vi "main_array.vi"() -> ()   [LabVIEW 2017]
panel:
  out "Numeric":i32
  out "error out":errorcluster
  in  "stop":bool
  in  "Mode":T1(tab)
  out "Polar Plot":picture
  in  "Plot Color":u32(colorbox)=16715776
  in  "Grid Color":u32(colorbox)
  in  "Visible Section":u16(ring)=8
  out "Range":dbl(slide) scale=0.0..600.0
  out "Histogram":picture
  in  "Clear":bool
  out "Array":i32[](array[numeric])
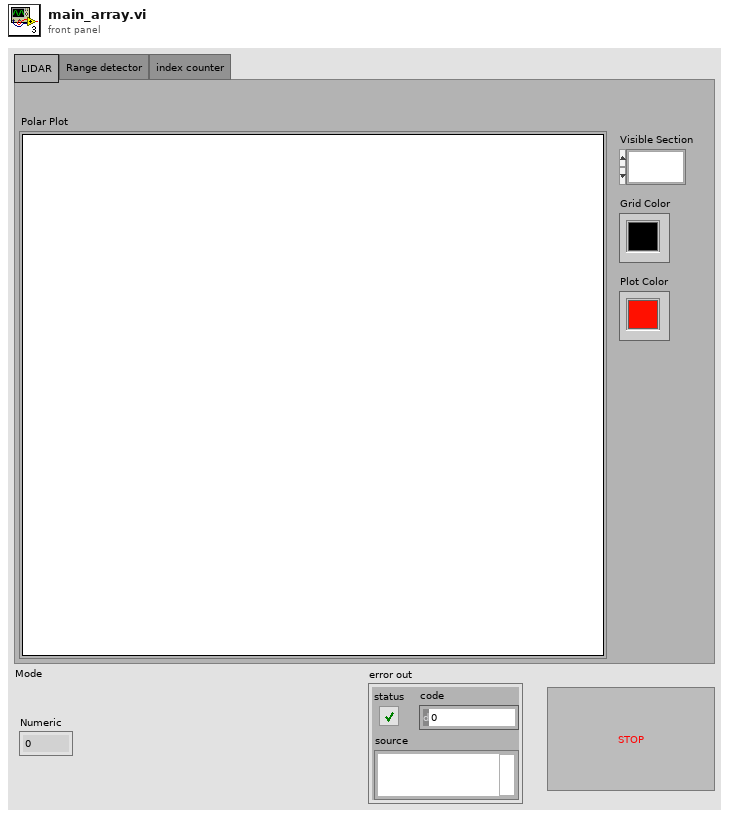
[diagram p1: front panel]
types:
  T1 = enum32{"LIDAR", "Range detector", "index counter"}
  T2 = cluster{"maximum":dbl, "minimum":dbl, "clip to min":bool, "log?(F)":bool, "grid color":u32, "plot color":u32, "format and precision":cluster{"format":enum8{"Decimal", "Scientific", "Engineering", "Binary", "Octal", "Hex"}, "precision":u8}, "visible section":u16}
  T3 = typedef "LVBoundsTypeDef.ctl" = cluster{"Width":u32, "Height":u32}
  T4 = cluster{"distance (C/AI0 (AI0))":dbl, "Numeric":dbl}
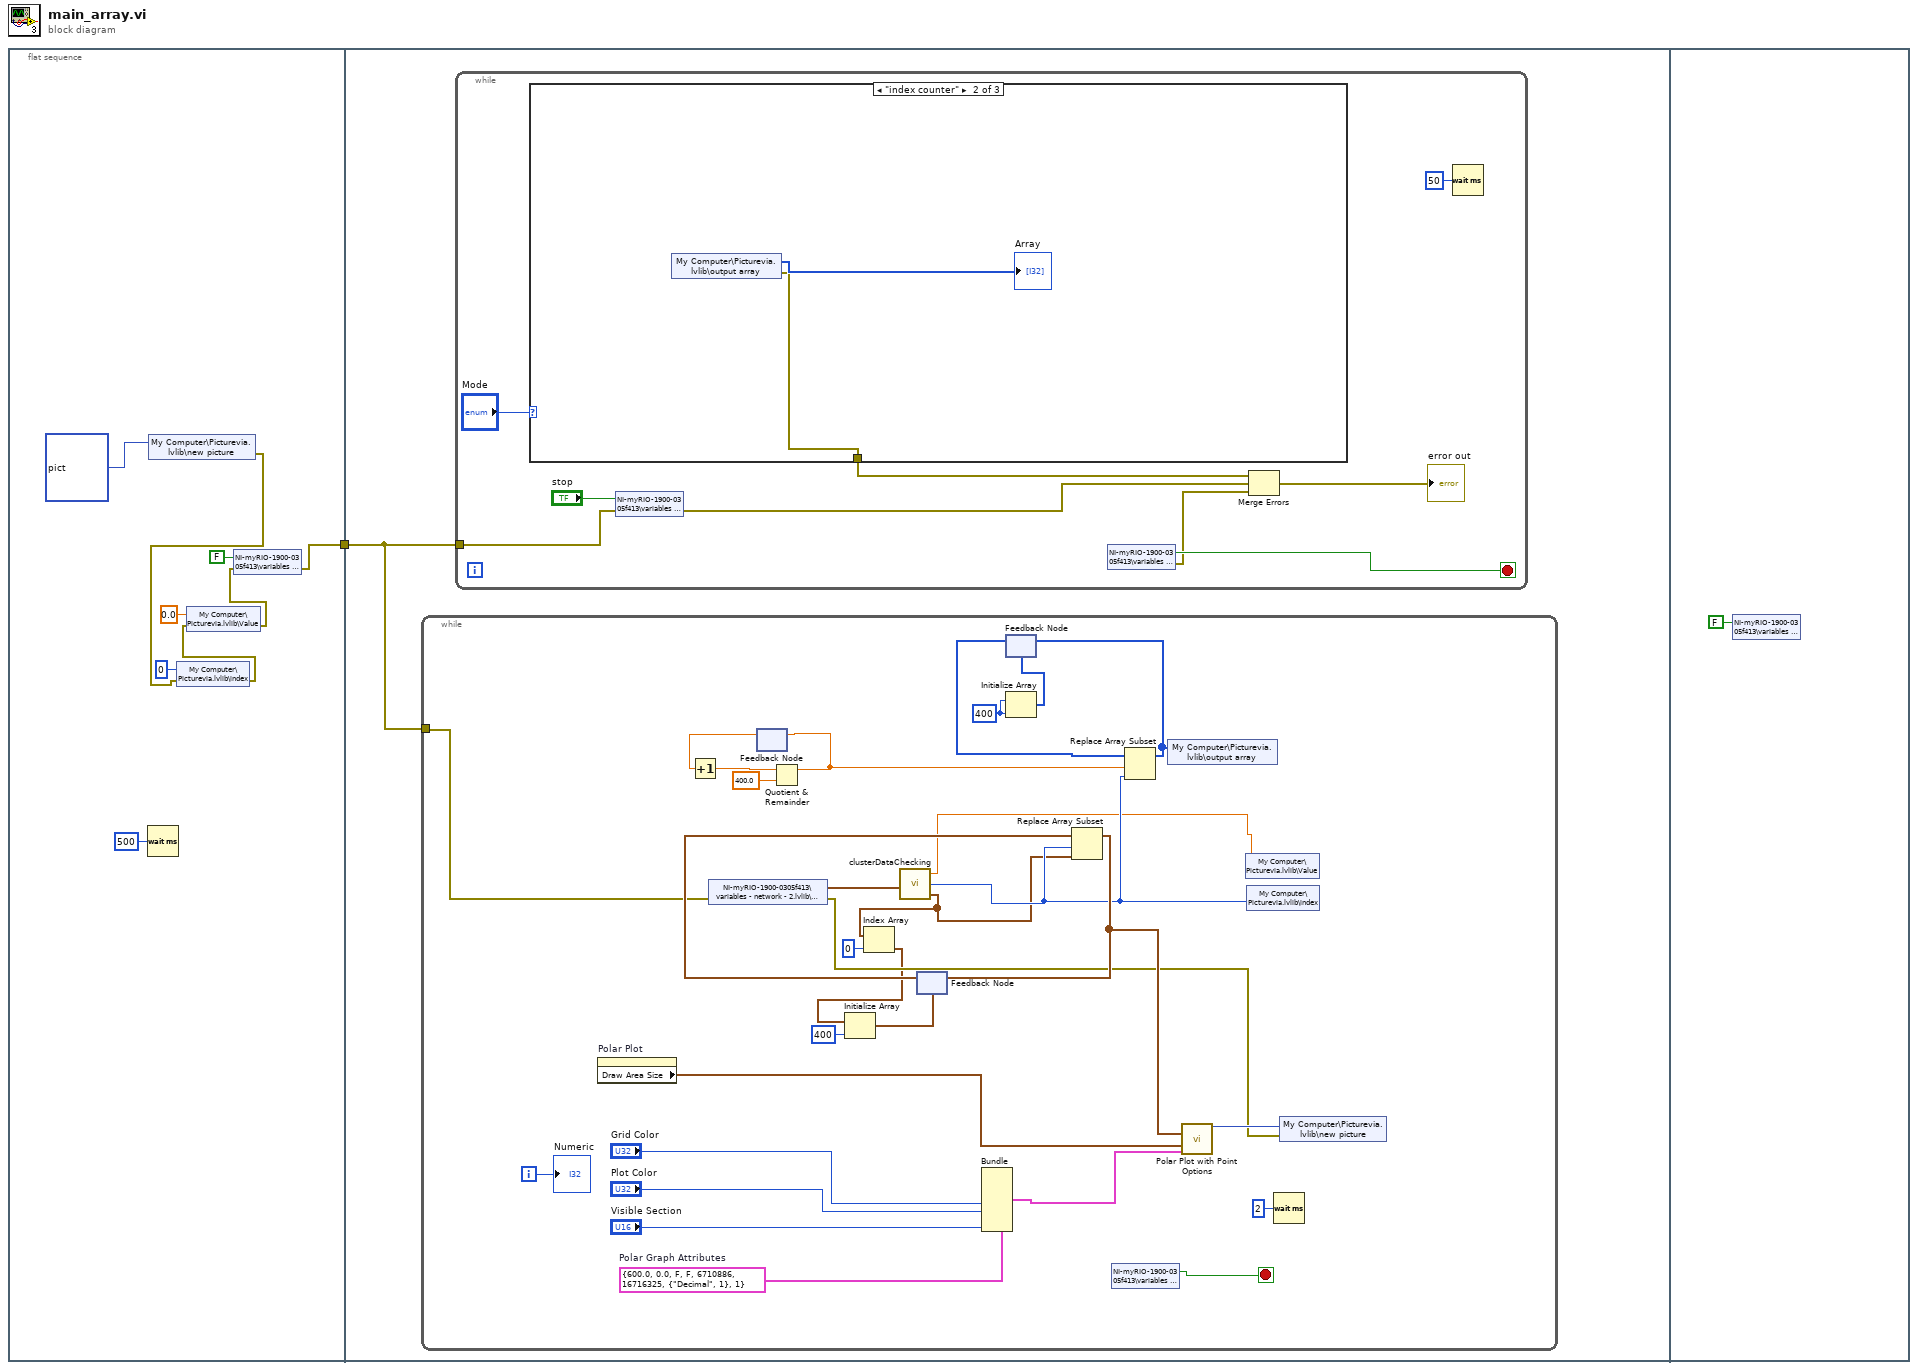
[diagram p0: block diagram]
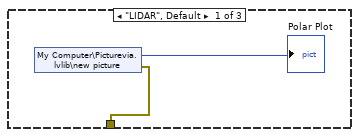
[diagram p2: hidden frame]
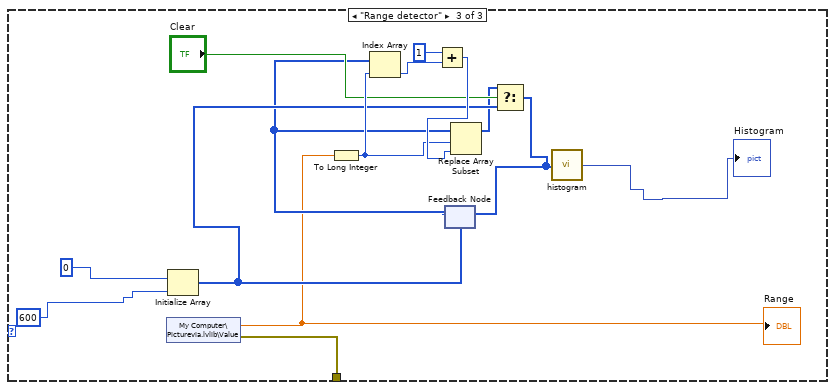
[diagram p3: hidden frame]
diagram:
  n1 = flat-sequence {
    tunnel: [w9] -> w1
    tunnel: w1 -> [w11]
    frame #0 {
      n2 = Wait (ms)(milliseconds to wait=u32 500) -> ()  [unwired: 1 out]
      n3 = shared-variable "My Computer\\Picturevia.lvlib\\new picture"(picture data[5B] ("new picture")) -> (error out=w3:errorcluster)  [unwired: 1 in]
      n4 = shared-variable "My Computer\\Picturevia.lvlib\\index"(0 ("index"), error in=w3) -> (error out=w6:errorcluster)
      n5 = shared-variable "My Computer\\Picturevia.lvlib\\Value"(0.0 ("Value"), error in=w6) -> (error out=w5:errorcluster)
      n6 = shared-variable "NI-myRIO-1900-0305f413\\variables - network - RT.lvlib\\stop"(FALSE ("stop"), error in=w5) -> (error out=w9:errorcluster)
    }
    frame #1 {
      n7 = while {
        tunnel: w11 -> [w26]
        i -> [w27]
        stop <- w29 stop-if-true
        w22 = 400 ("dimension size")
        w40 = T2 {"maximum"=600.0, "minimum"=0.0, "clip to min"=FALSE, "log?(F)"=FALSE, "grid color"=6710886, "plot color"=16716325, "format and precision"={"format"=enum."Decimal", "precision"=1}, "visible section"=1}  # Polar Graph Attributes
        n8 = property on="Polar Plot" class="Pict"() -> ("Draw Area Size"=w41:T3)  [unwired: 2 in, 2 out]
        n9 = shared-variable "NI-myRIO-1900-0305f413\\variables - network - 2.lvlib\\output cluster"(error in=w26) -> (w17:T4, error out=w30:errorcluster)
        n10 = feedback #1() -> (w19:dbl)  [unwired: 1 in]
        n11 = Increment(x=w19) -> (x+1=w21:dbl)
        n12 = Quotient & Remainder(x=w21, y=400.0) -> (x-y*floor(x/y)=w18:dbl)  [unwired: 1 out]
        n13 = feedback-in #1(w18) -> ()
        n14 = call "clusterDataChecking.vi"("Cluster input"=w17) -> ("value output"=w15:dbl, "index output"=w16:i32, "Array"=w14:cluster{"Numeric 2":dbl, dbl}[])
        n15 = Index Array(array=w14, index=0) -> (element=w12:cluster{"Numeric 2":dbl, dbl})
        n16 = Initialize Array(w12, 400 ("dimension size")) -> (w33:cluster{"Numeric 2":dbl, dbl}[])
        n17 = feedback #2(w33) -> (w35:cluster{"Numeric 2":dbl, dbl}[])
        n18 = Bundle(cluster=w40, "grid color"="Grid Color", "plot color"="Plot Color", "visible section"="Visible Section") -> (w32:T2)  [unwired: 5 in]
        n19 = Initialize Array(w22, w22) -> (w23:i32[])
        n20 = feedback #3(w23) -> (w24:i32[])
        n21 = Replace Array Subset(array=w35, new element=w14, index=w16) -> (w36:cluster{"Numeric 2":dbl, dbl}[])
        n22 = feedback-in #2(w36) -> ()
        n23 = shared-variable "NI-myRIO-1900-0305f413\\variables - network - RT.lvlib\\stop"() -> (w29:bool)  [unwired: 1 in, 1 out]
        n24 = Replace Array Subset(array=w24, new element=w16, index=w18) -> (w25:i32[])
        n25 = feedback-in #3(w25) -> ()
        n26 = shared-variable "My Computer\\Picturevia.lvlib\\output array"(w25) -> ()  [unwired: 1 in, 1 out]
        n27 = call <vilib>:"Polar Plot with Point Options.vi"("data array [mag, phase (deg)]"=w36, "dimensions (w,h)"=w41, "polar attributes"=w32) -> ("new picture"=w31:picture)  [unwired: 12 in]
        n28 = shared-variable "My Computer\\Picturevia.lvlib\\Value"(w15) -> ()  [unwired: 1 in, 1 out]
        n29 = shared-variable "My Computer\\Picturevia.lvlib\\index"(w16) -> ()  [unwired: 1 in, 1 out]
        n30 = Wait (ms)(milliseconds to wait=u32 2) -> ()  [unwired: 1 out]
        n31 = shared-variable "My Computer\\Picturevia.lvlib\\new picture"(w31, error in=w30) -> ()  [unwired: 1 out]
        "Numeric" <- w27
      }
      n32 = while {
        tunnel: w11 -> [w42]
        stop <- w44 stop-if-true
        n33 = case shown="\"index counter\"" "Mode" {
          tunnel: [w51 w53 w68] -> w46
          frame "LIDAR", Default {
            n34 = shared-variable "My Computer\\Picturevia.lvlib\\new picture"() -> (→"Polar Plot":picture, error out=w51:errorcluster)  [unwired: 1 in]
          }
          frame "index counter" {
            n35 = shared-variable "My Computer\\Picturevia.lvlib\\output array"() -> (→"Array":i32[], error out=w53:errorcluster)  [unwired: 1 in]
          }
          frame "Range detector" {
            n36 = shared-variable "My Computer\\Picturevia.lvlib\\Value"() -> (w56:dbl, error out=w68:errorcluster)  [unwired: 1 in]
            "Range" <- w56
            n37 = Initialize Array(0 ("element"), 600 ("dimension size")) -> (w61:i32[])
            n38 = To Long Integer(number=w56) -> (32bit integer=w63:i32)
            n39 = feedback #4(w61) -> (w59:i32[])
            n40 = Index Array(array=w59, index=w63) -> (element=w66:i32)
            n41 = Add(x=1, y=w66) -> (x+y=w65:i32)
            n42 = Replace Array Subset(array=w59, new element=w65, index=w63) -> (w58:i32[])
            n43 = Select(t=w58, s="Clear", f=w61) -> (s? t:f=w57:i32[])
            n44 = feedback-in #4(w57) -> ()
            n45 = call "histogram.vi"("Array"=w57) -> ("Histogram"=→"Histogram":picture)
          }
        }
        n46 = shared-variable "NI-myRIO-1900-0305f413\\variables - network - RT.lvlib\\stop"("stop", error in=w42) -> (error out=w49:errorcluster)
        n47 = shared-variable "NI-myRIO-1900-0305f413\\variables - network - RT.lvlib\\stop"() -> (w44:bool, error out=w43:errorcluster)  [unwired: 1 in]
        n48 = Merge Errors(w46, w49, w43) -> (→"error out":errorcluster)
        n49 = Wait (ms)(milliseconds to wait=u32 50) -> ()  [unwired: 1 out]
      }
    }
    frame #2 {
      n50 = shared-variable "NI-myRIO-1900-0305f413\\variables - network - RT.lvlib\\stop"(FALSE ("stop")) -> ()  [unwired: 1 in, 1 out]
    }
  }
